vi "Refresh Files Info.vi"(8 "error in (no error)":errorcluster, 11 "Session in":refnum<class "Session.lvclass">) -> (0 "error out":errorcluster, 3 "Session out":refnum<class "Session.lvclass">)   [LabVIEW 2020, in "Save for Previous Version.lvlib" / "Session.lvclass"]
uses:
  Session.lvclass
  Session.lvclass/Session.ctl
  File/File.lvclass/File.lvclass
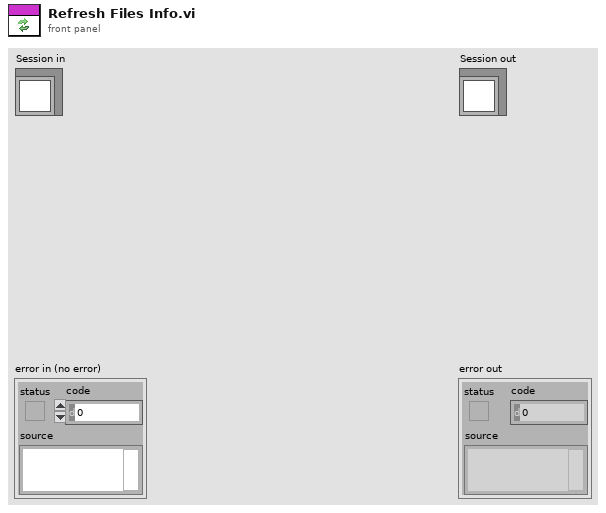
[diagram p1: front panel]
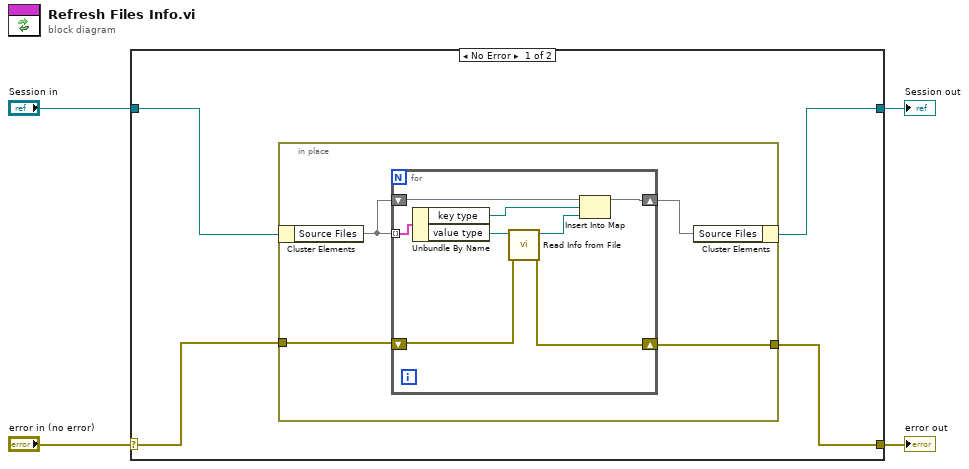
[diagram p0: block diagram]
diagram:
  n1 = case shown="No Error" "error in (no error)" {
    selector: "error in (no error)" -> [w8 w22]
    tunnel: [w7 w22] -> w3
    tunnel: [w6 w21] -> w1
    tunnel: "Session in" -> [w5 w21]
    frame No Error {
      n2 = in-place {
        in-place-border: w8 -> [w12]
        in-place-border: [w11] -> w7
        n3 = in-place-cluster #1(w5) -> ("Source Files"=w10:map{path, refnum<class "File.lvclass">})
        n4 = for {
          tunnel: w10 -> [w20] mode=indexing
          shift-right: [w18] -> w11
          shift-left: w12 -> [w19]
          shift-right: [w16] -> w9
          shift-left: w10 -> [w15]
          n5 = Unbundle By Name(w20) -> ("key type"=w14:path, "value type"=w17:refnum<class "File.lvclass">)
          n6 = call-dynamic "Read Info from File.vi"("error in (no error)"=w19, "File in"=w17) -> ("error out"=w18:errorcluster, "File out"=w13:refnum<class "File.lvclass">)  [unwired: 8 in]
          n7 = Insert Into Map(map in=w15, key=w14, value=w13) -> (map out=w16:map{path, refnum<class "File.lvclass">})  [unwired: 2 out]
        }
        n8 = in-place-cluster #1("Source Files"=w9) -> (w6:refnum<class "Session.lvclass">)
      }
    }
    frame Error {
    }
  }
  "error out" <- w3
  "Session out" <- w1
